vi "CompensateXY.vi"(1 "Inverse Matrix":T2, 2 "Current Data":T1, 3 "Target Found?":bool, 4 "Target Data":T1) -> (0 "XY Displacement":dbl[](array[numeric]))   [LabVIEW 2014]
uses:
  <vilib>/Analysis/Matrix/Datatypes/RealMatrix.ctl
  <vilib>/Analysis/baseanly.llb/A x Vector.vi
  <vilib>/Analysis/NI_AALBase.lvlib
  <vilib>/Analysis/Matrix/NI_Matrix.lvlib
panel:
  # "LICENSED MATERIALS – PROPERTY OF IBM\nCopyright IBM Corp. 2016,\nALL RIGHTS RESERVED"
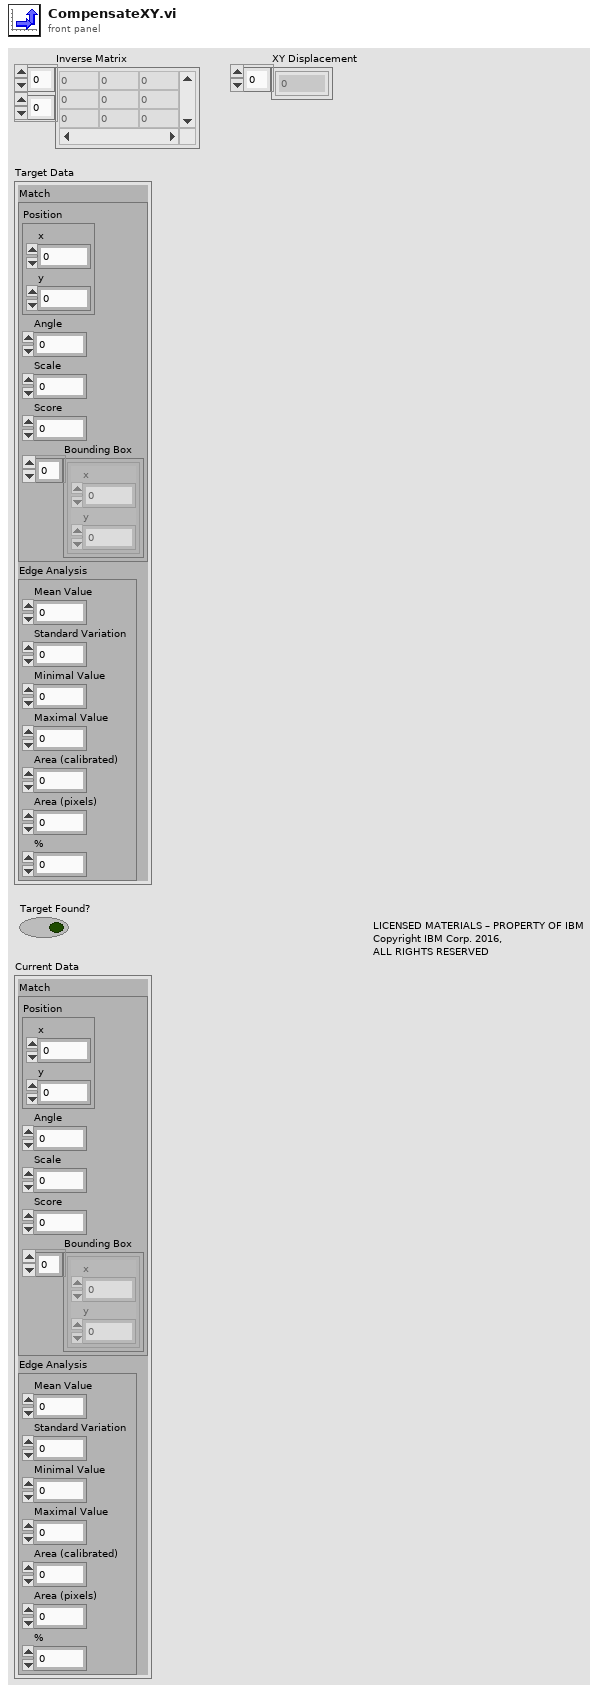
[diagram p1: front panel]
types:
  T1 = cluster{"Match":cluster{"Position":cluster{"x":sgl, "y":sgl}, "Angle":sgl, "Scale":sgl, "Score":sgl, "Bounding Box":cluster{"x":sgl, "y":sgl}[]}, "Edge Analysis":cluster{"Mean Value":sgl, "Standard Variation":sgl, "Minimal Value":sgl, "Maximal Value":sgl, "Area (calibrated)":sgl, "Area (pixels)":i32, "%":sgl}}
  T2 = typedef "NI_Matrix.lvlib/RealMatrix.ctl" = dbl[][]
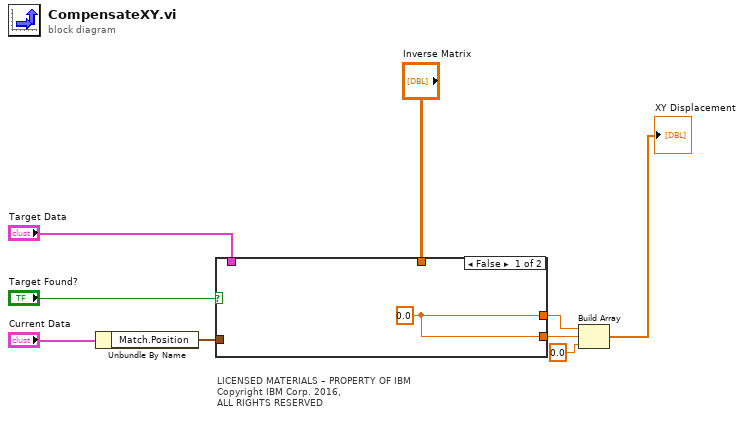
[diagram p0: block diagram]
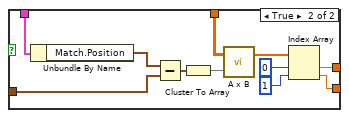
[diagram p2: hidden frame]
diagram:
  # "LICENSED MATERIALS – PROPERTY OF IBM\nCopyright IBM Corp. 2016,\nALL RIGHTS RESERVED"
  n1 = Unbundle By Name("Current Data") -> ("Match.Position"=w1:cluster{"x":sgl, "y":sgl})
  n2 = case shown="False" "Target Found?" {
    tunnel: w1 -> [_ w11]
    tunnel: "Target Data" -> [_ w16]
    tunnel: [w10 w15] -> w4
    tunnel: [w10 w14] -> w5
    tunnel: "Inverse Matrix" -> [_ w13]
    frame False {
      w10 = 0.0
    }
    frame True {
      n3 = Unbundle By Name(w16) -> ("Match.Position"=w12:cluster{"x":sgl, "y":sgl})
      n4 = Subtract(x=w12, y=w11) -> (x-y=w18:cluster{"x":sgl, "y":sgl})
      n5 = Cluster To Array(cluster=w18) -> (array=w17:sgl[])
      n6 = call-poly <vilib>:"A x B.vi"("Vector"=w17, "A"=w13) -> ("A x Vector"=w21:dbl[])  [unwired: 1 out]
      n7 = Index Array(array=w21, index #1=0 ("index"), index #2=1 ("index")) -> (element #1=w15:dbl, element #2=w14:dbl)
    }
  }
  n8 = Build Array(w4, w5, 0.0 ("element")) -> (→"XY Displacement":dbl[])
